vi "Process.vi"(8 "error in (no error)":errorcluster, 10 "Pound":refnum<class "Pound.lvclass">, 11 "Qbus in":refnum<class "Qbus.lvclass">) -> (0 "error out":errorcluster)   [LabVIEW 2017, in "BlinkProcess.lvlib"]
doc: "Controls the blink behavior of the USER1 LED on the front panel of a CompactRIO controller."
uses:
  <vilib>/addons/BlinkProcess/BlinkProcess.lvlib
  <vilib>/addons/Qbus/Qbus.lvclass
  <vilib>/NI/Software Watchdog/Pound/Pound.lvclass
  <vilib>/addons/BlinkProcess/controls/ModeConfig.ctl
  <vilib>/addons/BlinkProcess/controls/mode.ctl
  <vilib>/addons/BlinkProcess/controls/customBlinkConfig.ctl
  <vilib>/NI/Software Watchdog/Watchdog/Watchdog.lvclass
panel:
  out "Led State":bool
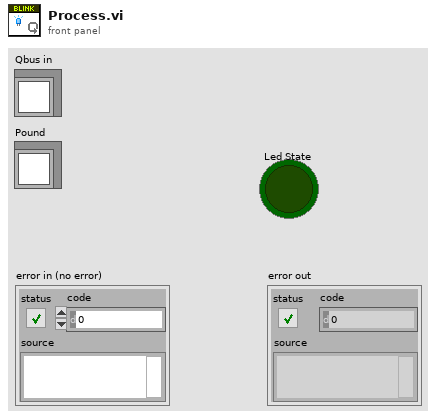
[diagram p1: front panel]
types:
  T1 = typedef "BlinkProcess.lvlib/ModeConfig.ctl" = cluster{"mode":T2, "custom blink":T3}
  T2 = typedef "BlinkProcess.lvlib/mode.ctl" = enum16{"Normal", "Error", "On", "Off", "Custom"}
  T3 = typedef "BlinkProcess.lvlib/customBlinkConfig.ctl" = cluster{"pattern rate (sec)":dbl, "number of blinks":u32}
  T4 = typedef "BlinkProcess.lvlib/CustomBlinkInternalState.ctl" = cluster{"period":i32, "transitions":i32[]}
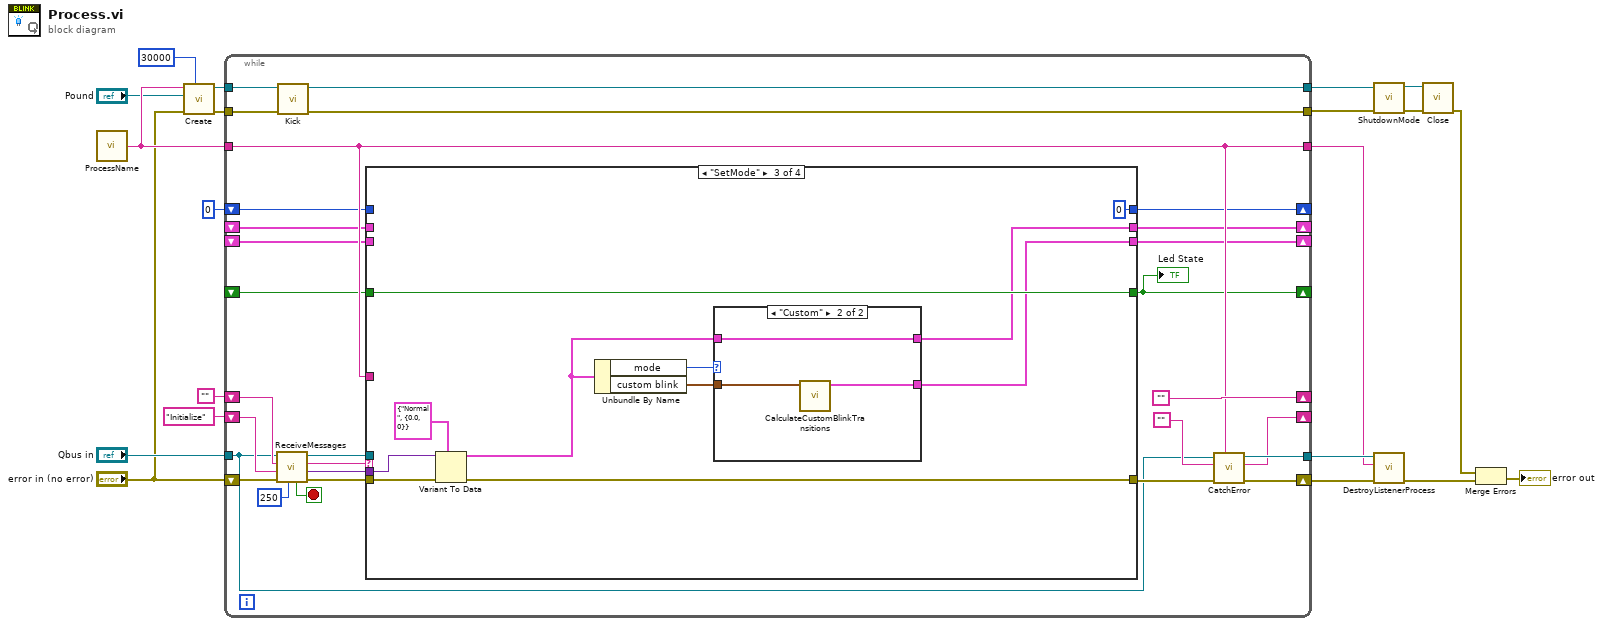
[diagram p0: block diagram]
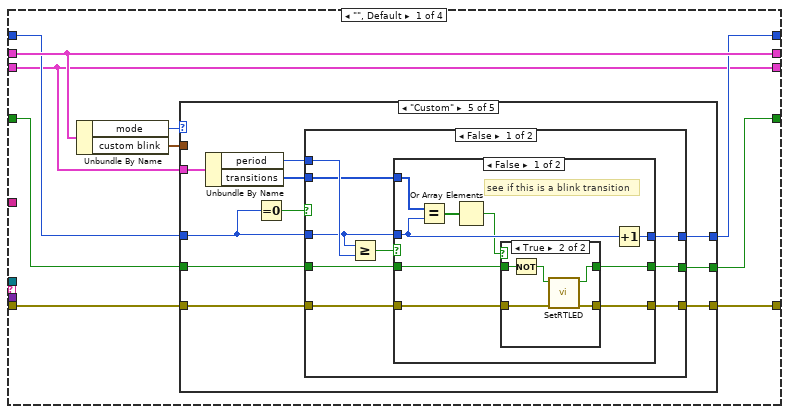
[diagram p2: hidden frame]
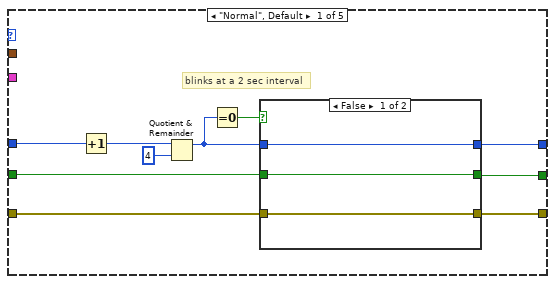
[diagram p3: hidden frame]
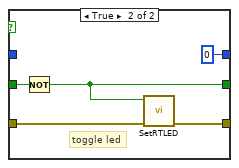
[diagram p4: hidden frame]
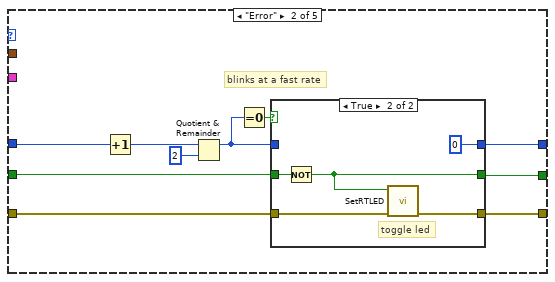
[diagram p5: hidden frame]
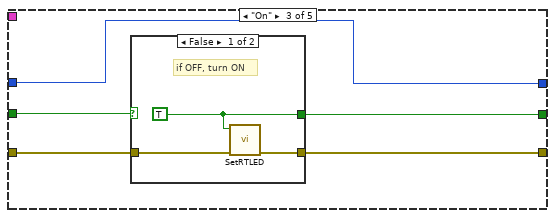
[diagram p7: hidden frame]
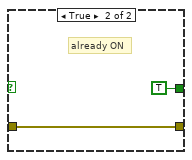
[diagram p8: hidden frame]
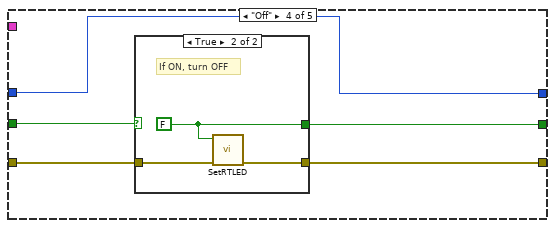
[diagram p9: hidden frame]
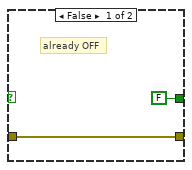
[diagram p10: hidden frame]
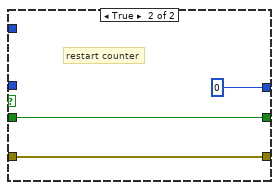
[diagram p12: hidden frame]
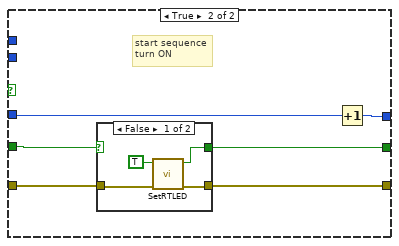
[diagram p13: hidden frame]
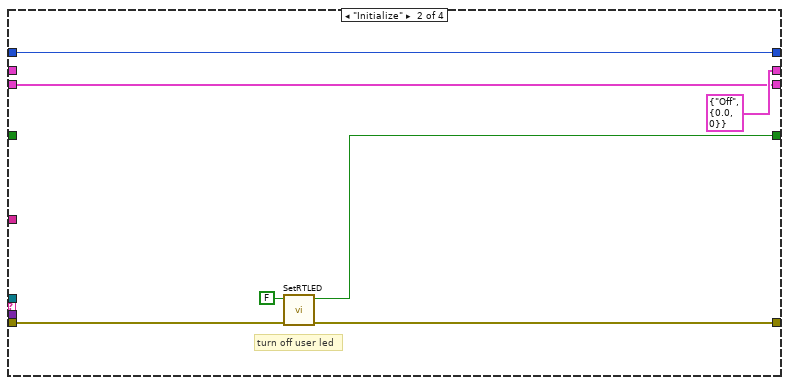
[diagram p15: hidden frame]
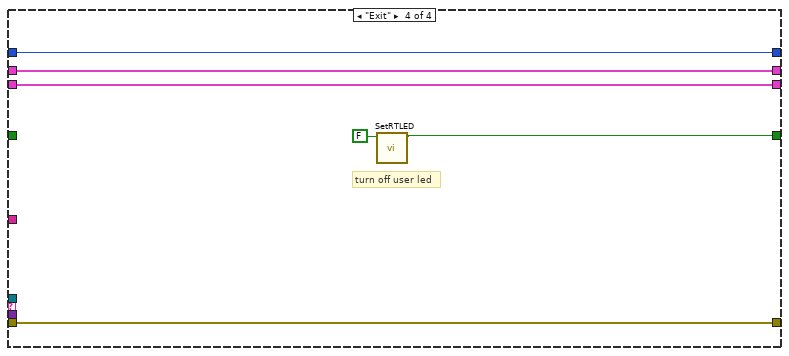
[diagram p17: hidden frame]
diagram:
  n1 = call <vilib>:"ProcessName.vi"() -> ("process name"=w13:string)  [unwired: 5 in]
  n2 = call <vilib>:"Create.vi"("Execution Timeout (ms)"=u32 30000, "error in (no error)"="error in (no error)", "Pound"="Pound", "Name"=w13) -> ("error out"=w10:errorcluster, "Watchdog"=w11:refnum<data-value>)  [unwired: 6 in]
  n3 = while {
    shift-right: [""] -> _
    shift-left: "" -> [w47]
    tunnel: "Qbus in" -> [w21]
    tunnel: w13 -> [w37]
    tunnel: [w40] -> w18
    tunnel: [w37] -> w17
    shift-right: [w38] -> _
    shift-left: "Initialize" -> [w42]
    shift-right: [w36] -> _
    shift-left: _ -> [w35]
    shift-right: [w31] -> _
    shift-left: 0 -> [w34]
    shift-right: [w33] -> _
    shift-left: _ -> [w32]
    tunnel: w11 -> [w30]
    tunnel: w10 -> [w29]
    tunnel: [w28] -> w6
    tunnel: [w27] -> w7
    shift-right: [w26] -> _
    shift-left: _ -> [w25]
    shift-right: [w41] -> w19
    shift-left: "error in (no error)" -> [w49]
    stop <- w48 stop-if-true
    n4 = call <vilib>:"ReceiveMessages.vi"("timeout(100)"=250 ("Timeout(100)"), "error in (no error)"=w49, "priority action"=w42, "default action"=w47, "Qbus in"=w21) -> ("error out"=w46:errorcluster, "message value"=w43:variant, "action"=w24:string, "Qbus out"=w44:refnum<class "Qbus.lvclass">, "exit"=w48:bool)  [unwired: 2 in]
    n5 = call <vilib>:"Kick.vi"("error in (no error)"=w29, "Watchdog"=w30) -> ("error out"=w27:errorcluster, "Watchdog"=w28:refnum<data-value>)  [unwired: 8 in]
    n6 = case shown="\"SetMode\"" w24 {
      tunnel: w46 -> [w59 w166 w183 w193]
      tunnel: w44 -> [_ _ _ _]
      tunnel: [w58 w169 w181 w193] -> w22
      tunnel: w43 -> [_ _ w182 _]
      tunnel: w37 -> [_ _ _ _]
      tunnel: [w56 w170 w179 w189] -> w36
      tunnel: w35 -> [w57 _ w179 _]
      tunnel: w34 -> [w52 w172 _ w191]
      tunnel: [w54 T1 {"mode"=enum."Off", "custom blink"={"pattern rate (sec)"=0.0, "number of blinks"=0}} ("Mode Config") w175 w192] -> w33
      tunnel: w32 -> [w54 _ _ w192]
      tunnel: [w51 w172 0 w191] -> w31
      tunnel: [w50 w167 w174 w188] -> w26
      tunnel: w25 -> [w50 w167 _ w188]
      frame "", Default {
        n7 = Unbundle By Name(w54) -> ("mode"=w55:T2, "custom blink"=w53:T3)
        n8 = case shown="\"Custom\"" w55 {
          tunnel: w59 -> [w69 w87 w100 w110 w122]
          tunnel: w57 -> [w65 w83 w97 w107 w123]
          tunnel: [w68 w86 w99 w109 w121] -> w58
          tunnel: [w63 w81 w96 w106 w116] -> w51
          tunnel: [w62 w80 w98 w108 w120] -> w56
          tunnel: w53 -> [_ _ _ _ _]
          tunnel: w52 -> [w61 w79 w96 w106 w117]
          tunnel: w50 -> [_ _ _ _ w125]
          frame "Normal", Default {
            # "blinks at a 2 sec interval"
            n9 = Increment(x=w61) -> (x+1=w60:i32)
            n10 = Quotient & Remainder(x=w60, y=4) -> (x-y*floor(x/y)=w64:i32)  [unwired: 1 out]
            n11 = Equal To 0?(x=w64) -> (x = 0?=w66:bool)
            n12 = case shown="False" w66 {
              tunnel: w69 -> [w71 w74]
              tunnel: [w71 w75] -> w68
              tunnel: w65 -> [w70 w76]
              tunnel: w64 -> [w72 _]
              tunnel: [w72 0] -> w63
              tunnel: [w70 w73] -> w62
              frame False {
              }
              frame True {
                # "toggle led"
                n13 = Not(x=w76) -> (.not. x?=w73:bool)
                n14 = call <vilib>:"SetRTLED.vi"("error in (no error)"=w74, "LED state"=w73) -> ("error out"=w75:errorcluster)  [unwired: 8 in, 1 out]
              }
            }
          }
          frame "Error" {
            # "blinks at a fast rate"
            n15 = Increment(x=w79) -> (x+1=w78:i32)
            n16 = Quotient & Remainder(x=w78, y=2) -> (x-y*floor(x/y)=w82:i32)  [unwired: 1 out]
            n17 = Equal To 0?(x=w82) -> (x = 0?=w84:bool)
            n18 = case shown="True" w84 {
              tunnel: w87 -> [w89 w93]
              tunnel: [w89 w91] -> w86
              tunnel: w83 -> [w88 w94]
              tunnel: w82 -> [w90 _]
              tunnel: [w90 0] -> w81
              tunnel: [w88 w92] -> w80
              frame False {
              }
              frame True {
                # "toggle led"
                n19 = Not(x=w94) -> (.not. x?=w92:bool)
                n20 = call <vilib>:"SetRTLED.vi"("error in (no error)"=w93, "LED state"=w92) -> ("error out"=w91:errorcluster)  [unwired: 8 in, 1 out]
              }
            }
          }
          frame "On" {
            n21 = case shown="False" w97 {
              tunnel: w100 -> [w103 w105]
              tunnel: [w102 w105] -> w99
              tunnel: [w101 TRUE] -> w98
              frame False {
                w101 = TRUE
                # "if OFF, turn ON"
                n22 = call <vilib>:"SetRTLED.vi"("error in (no error)"=w103, "LED state"=w101) -> ("error out"=w102:errorcluster)  [unwired: 8 in, 1 out]
              }
              frame True {
                # "already ON"
              }
            }
          }
          frame "Off" {
            n23 = case shown="True" w107 {
              tunnel: w110 -> [w112 w115]
              tunnel: [w112 w114] -> w109
              tunnel: [FALSE w113] -> w108
              frame False {
                # "already OFF"
              }
              frame True {
                w113 = FALSE
                # "If ON, turn OFF"
                n24 = call <vilib>:"SetRTLED.vi"("error in (no error)"=w115, "LED state"=w113) -> ("error out"=w114:errorcluster)  [unwired: 8 in, 1 out]
              }
            }
          }
          frame "Custom" {
            n25 = Unbundle By Name(w125) -> ("period"=w119:i32, "transitions"=w118:i32[])
            n26 = Equal To 0?(x=w117) -> (x = 0?=w124:bool)
            n27 = case shown="False" w124 {
              tunnel: w123 -> [w129 w159]
              tunnel: w122 -> [w130 w158]
              tunnel: [w127 w157] -> w121
              tunnel: [w128 w156] -> w120
              tunnel: w119 -> [w134 _]
              tunnel: w118 -> [w126 _]
              tunnel: w117 -> [w132 w154]
              tunnel: [w131 w155] -> w116
              frame False {
                n28 = Greater Or Equal?(x=w132, y=w134) -> (x >= y?=w133:bool)
                n29 = case shown="False" w133 {
                  tunnel: w132 -> [w140 _]
                  tunnel: [w141 0] -> w131
                  tunnel: w130 -> [w138 w151]
                  tunnel: w129 -> [w135 w152]
                  tunnel: [w137 w152] -> w128
                  tunnel: [w136 w151] -> w127
                  tunnel: w126 -> [w143 _]
                  frame False {
                    # "see if this is a blink transition"
                    n30 = Equal?(x=w143, y=w140) -> (x = y?=w142:bool[])
                    n31 = Or Array Elements(Boolean array=w142) -> (logical OR=w139:bool)
                    n32 = case shown="True" w139 {
                      tunnel: w138 -> [w144 w150]
                      tunnel: [w145 w148] -> w137
                      tunnel: [w144 w147] -> w136
                      tunnel: w135 -> [w145 w146]
                      frame False {
                      }
                      frame True {
                        n33 = Not(x=w146) -> (.not. x?=w149:bool)
                        n34 = call <vilib>:"SetRTLED.vi"("error in (no error)"=w150, "LED state"=w149) -> ("error out"=w147:errorcluster, "LED state"=w148:bool)  [unwired: 8 in]
                      }
                    }
                    n35 = Increment(x=w140) -> (x+1=w141:i32)
                  }
                  frame True {
                    # "restart counter"
                  }
                }
              }
              frame True {
                # "start sequence\nturn ON"
                n36 = case shown="False" w159 {
                  selector: w159 -> [_ w164]
                  tunnel: w158 -> [w160 w165]
                  tunnel: [w163 w165] -> w157
                  tunnel: [w161 w164] -> w156
                  frame False {
                    n37 = call <vilib>:"SetRTLED.vi"("error in (no error)"=w160, "LED state"=TRUE) -> ("error out"=w163:errorcluster, "LED state"=w161:bool)  [unwired: 8 in]
                  }
                  frame True {
                  }
                }
                n38 = Increment(x=w154) -> (x+1=w155:i32)
              }
            }
          }
        }
      }
      frame "Initialize" {
        # "turn off user led"
        n39 = call <vilib>:"SetRTLED.vi"("error in (no error)"=w166, "LED state"=FALSE) -> ("error out"=w169:errorcluster, "LED state"=w170:bool)  [unwired: 8 in]
      }
      frame "SetMode" {
        n40 = Variant To Data(error in=w183, type=T1 {"mode"=enum."Normal", "custom blink"={"pattern rate (sec)"=0.0, "number of blinks"=0}} ("Mode Config"), Variant=w182) -> (data=w176:T1, error out=w181:errorcluster)
        n41 = Unbundle By Name(w176) -> ("mode"=w178:T2, "custom blink"=w177:T3)
        n42 = case shown="\"Custom\"" w178 {
          tunnel: w177 -> [_ w186]
          tunnel: w176 -> [w184 w187]
          tunnel: [w184 w187] -> w175
          tunnel: [_ w185] -> w174
          frame "Normal", Default {
          }
          frame "Custom" {
            n43 = call <vilib>:"CalculateCustomBlinkTransitions.vi"("custom blink"=w186) -> ("custom blink internal state"=w185:T4)  [unwired: 10 in]
          }
        }
      }
      frame "Exit" {
        # "turn off user led"
        n44 = call <vilib>:"SetRTLED.vi"("LED state"=FALSE) -> ("LED state"=w189:bool)  [unwired: 9 in, 1 out]
      }
    }
    "Led State" <- w36
    n45 = call <vilib>:"CatchError.vi"("source"=w37, "error in (no error)"=w22, "next action in"="", "Qbus in"=w21) -> ("error out"=w41:errorcluster, "next action out"=w38:string, "Qbus out"=w40:refnum<class "Qbus.lvclass">)  [unwired: 5 in]
  }
  n46 = call <vilib>:"ShutdownMode.vi"("error in (no error)"=w7, "Watchdog"=w6) -> ("error out"=w8:errorcluster, "Watchdog"=w9:refnum<data-value>)  [unwired: 8 in]
  n47 = call <vilib>:"DestroyListenerProcess.vi"("error in (no error)"=w19, "process name"=w17, "Qbus in"=w18) -> ("error in (no error)"=w4:errorcluster)  [unwired: 7 in, 1 out]
  n48 = call <vilib>:"Close.vi"("error in (no error)"=w8, "Watchdog"=w9) -> ("error out"=w5:errorcluster)  [unwired: 9 in]
  n49 = Merge Errors(w5, w4) -> (→"error out":errorcluster)
